vi "Register Core gRPC Server.vi"(8 "error in (no error)":errorcluster, 10 "gRPC ID":T1, 11 "CIFTemplateNode in":refnum<class "CIFCorePlugin.lvclass">) -> (0 "error out":errorcluster, 2 "gRPC ID Out":T1, 3 "CIFTemplateNode out":refnum<class "CIFCorePlugin.lvclass">)   [LabVIEW 2021, in "CIFCorePlugin.lvclass"]
uses:
  CIFCorePlugin.lvclass
  <vilib>/gRPC/LabVIEW gRPC Library/Shared/grpcId.ctl
  CIFCorePlugin.lvclass/CIFCorePlugin.ctl
  Grpc/CIFCorePlugin_server/RPC Service/PluginCore/PluginCore.lvclass
  C:/Program Files/National Instruments/LabVIEW 2021/vi.lib/gRPC/LabVIEW gRPC Servicer/ServiceBase/ServiceBase.lvclass
  Grpc/CIFCoreChannel_server/RPC Service/ChannelCore/ChannelCore.lvclass
  <vilib>/gRPC/LabVIEW gRPC Library/Server API/Server/Register Message Metadata.vi
  <vilib>/gRPC/LabVIEW gRPC Library/Server API/Server/Register Enum Metadata.vi
  Grpc/CIFCorePlugin_server/CIFCorePlugin_server.lvlib
  Grpc/CIFCoreChannel_server/CIFCoreChannel_server.lvlib
  <vilib>/gRPC/LabVIEW gRPC Library/grpc-lvsupport-release.lvlib
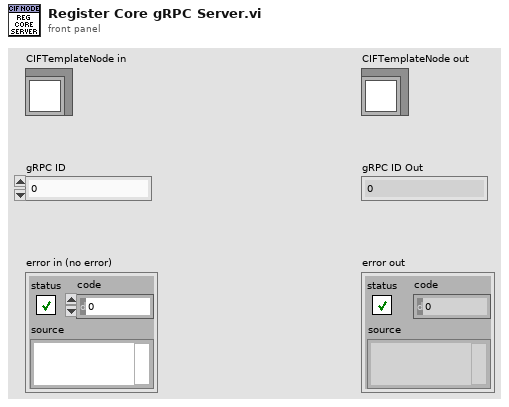
[diagram p1: front panel]
types:
  T1 = typedef "grpc-lvsupport-release.lvlib/grpcId.ctl" = u64
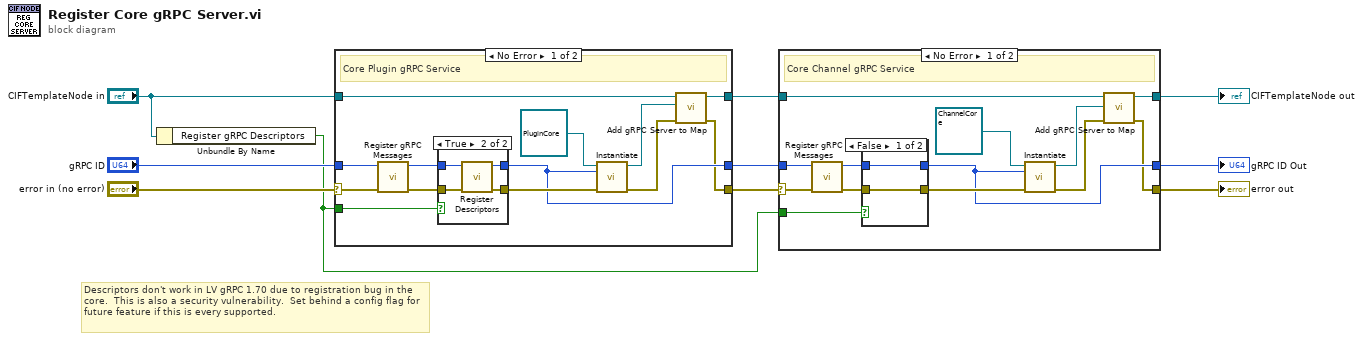
[diagram p0: block diagram]
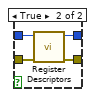
[diagram p2: hidden frame]
diagram:
  # "Descriptors don't work in LV gRPC 1.70 due to registration bug in the core.  This is also a security vulnerability.  Set behind a config flag for future feature if this is every supported."
  n1 = Unbundle By Name("CIFTemplateNode in") -> ("Register gRPC Descriptors"=w1:bool)
  n2 = case shown="No Error" "error in (no error)" {
    selector: "error in (no error)" -> [w21 w32]
    tunnel: [w12 w32] -> w7
    tunnel: [w17 w31] -> w8
    tunnel: "CIFTemplateNode in" -> [w18 w31]
    tunnel: "gRPC ID" -> [w20 w30]
    tunnel: [w13 w30] -> w6
    tunnel: w1 -> [w11 _]
    frame No Error {
      # "Core Plugin gRPC Service"
      n3 = call "Register gRPC Messages.vi"("error in (no error)"=w21, "gRPC ID"=w20) -> ("error out"=w22:errorcluster, "gRPC ID Out"=w23:T1)  [unwired: 8 in]
      n4 = case shown="True" w11 {
        tunnel: w23 -> [w25 w29]
        tunnel: w22 -> [w24 w28]
        tunnel: [w24 w27] -> w19
        tunnel: [w25 w26] -> w13
        frame False {
        }
        frame True {
          n5 = call "Register Descriptors.vi"("error in (no error)"=w28, "gRPC ID"=w29) -> ("error out"=w27:errorcluster, "gRPC ID Out"=w26:T1)  [unwired: 8 in]
        }
      }
      n6 = call-dynamic "Instantiate.vi"("error in"=w19, "gRPCid"=w13, "gRPC service in"=refnum<class "PluginCore.lvclass"> refnum ("CIF_Plugin_Core_server.lvlib:PluginCore.lvclass")) -> ("error out"=w15:errorcluster, "gRPC service out"=w14:refnum<class "PluginCore.lvclass">)  [unwired: 7 in]
      n7 = call "Add gRPC Server to Map.vi"("error in (no error)"=w15, "gRPC Server Class"=w14, "CIFTemplateNode in"=w18) -> ("error out"=w12:errorcluster, "CIFTemplateNode out"=w17:refnum<class "CIFCorePlugin.lvclass">)  [unwired: 7 in]
    }
    frame Error {
    }
  }
  n8 = case shown="No Error" w7 {
    selector: w7 -> [w43 w54]
    tunnel: [w36 w54] -> w3
    tunnel: [w39 w53] -> w4
    tunnel: w8 -> [w40 w53]
    tunnel: w6 -> [w42 w52]
    tunnel: [w37 w52] -> w5
    tunnel: w1 -> [w33 _]
    frame No Error {
      # "Core Channel gRPC Service"
      n9 = call "Register gRPC Messages.vi"("error in (no error)"=w43, "gRPC ID"=w42) -> ("error out"=w44:errorcluster, "gRPC ID Out"=w45:T1)  [unwired: 8 in]
      n10 = case shown="False" w33 {
        tunnel: w45 -> [w47 w51]
        tunnel: w44 -> [w46 w50]
        tunnel: [w46 w49] -> w41
        tunnel: [w47 w48] -> w37
        frame False {
        }
        frame True {
          n11 = call "Register Descriptors.vi"("error in (no error)"=w50, "gRPC ID"=w51) -> ("error out"=w49:errorcluster, "gRPC ID Out"=w48:T1)  [unwired: 8 in]
        }
      }
      n12 = call-dynamic "Instantiate.vi"("error in"=w41, "gRPCid"=w37, "gRPC service in"=refnum<class "ChannelCore.lvclass"> refnum ("CIFCoreChannel_server.lvlib:ChannelCore.lvclass")) -> ("error out"=w38:errorcluster, "gRPC service out"=w35:refnum<class "ChannelCore.lvclass">)  [unwired: 7 in]
      n13 = call "Add gRPC Server to Map.vi"("error in (no error)"=w38, "gRPC Server Class"=w35, "CIFTemplateNode in"=w40) -> ("error out"=w36:errorcluster, "CIFTemplateNode out"=w39:refnum<class "CIFCorePlugin.lvclass">)  [unwired: 7 in]
    }
    frame Error {
    }
  }
  "error out" <- w3
  "CIFTemplateNode out" <- w4
  "gRPC ID Out" <- w5
